vi "Set IPS120 Control.vi"(8 "Error In":errorcluster, 11 "VISA resource name":refnum<visa-resource-name>) -> (0 "Error Out":errorcluster, 3 "VISA resource name out":refnum<visa-resource-name>)   [LabVIEW 2018]
uses:
  Controls/Sweep Action.ctl
panel:
  in  "Command string":string
  in  "Sweep action":T1
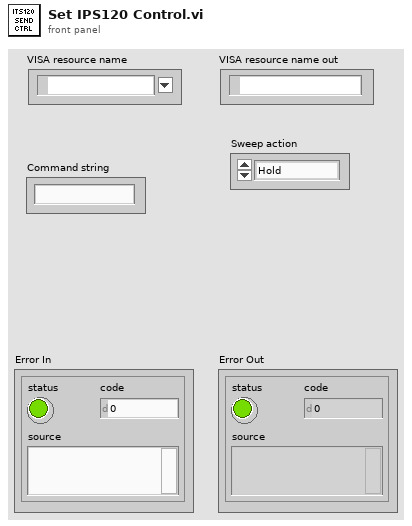
[diagram p1: front panel]
types:
  T1 = typedef "Sweep Action.ctl" = enum16{"Hold", "To set point", "To zero", "Clamp"}
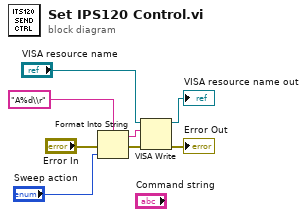
[diagram p0: block diagram]
diagram:
  n1 = Format Into String(format string="A%d\\r", error in="Error In", "Sweep action") -> (resulting string=w4:string, error out=w5:errorcluster)  [unwired: 1 in]
  n2 = VISA Write(VISA resource name="VISA resource name", write buffer=w4, error in (no error)=w5) -> (VISA resource name out=→"VISA resource name out":refnum<visa-resource-name>, error out=→"Error Out":errorcluster)  [unwired: 1 out]
